vi "DTMF.vi"() -> ()   [LabVIEW 2019]
uses:
  Control 1.ctl
  <vilib>/Waveform/WDTOps.llb/WDT Number of Waveform Samples DBL.vi
  <vilib>/Waveform/WDTOps.llb/WDT Get Waveform Subset DBL.vi
panel:
  out "size(s)":i32
  out "Waveform Chart":dynamicdata(graph)
  in  "stop":bool
  in  "Waveform":waveform(dbl)
  in  "Load File":bool
  out "String":string
  in  "Mode":bool
  out "Collected Signals":dynamicdata(graph)
  out "Signals":dynamicdata(graph)
  in  "stop (F)":bool
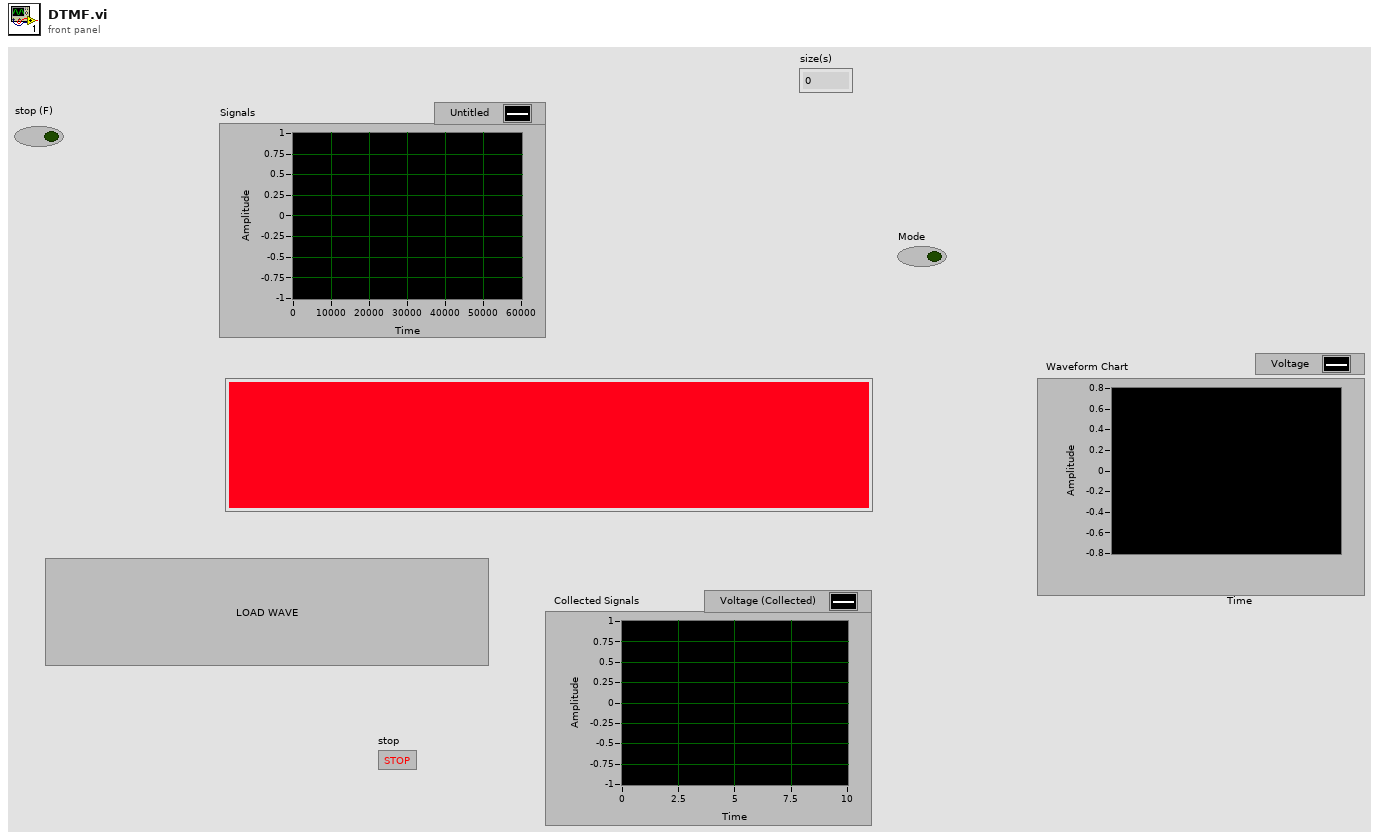
[diagram p1: front panel]
types:
  T1 = typedef "Control 1.ctl" = enum16{"Idle", "Load Image", "Process"}
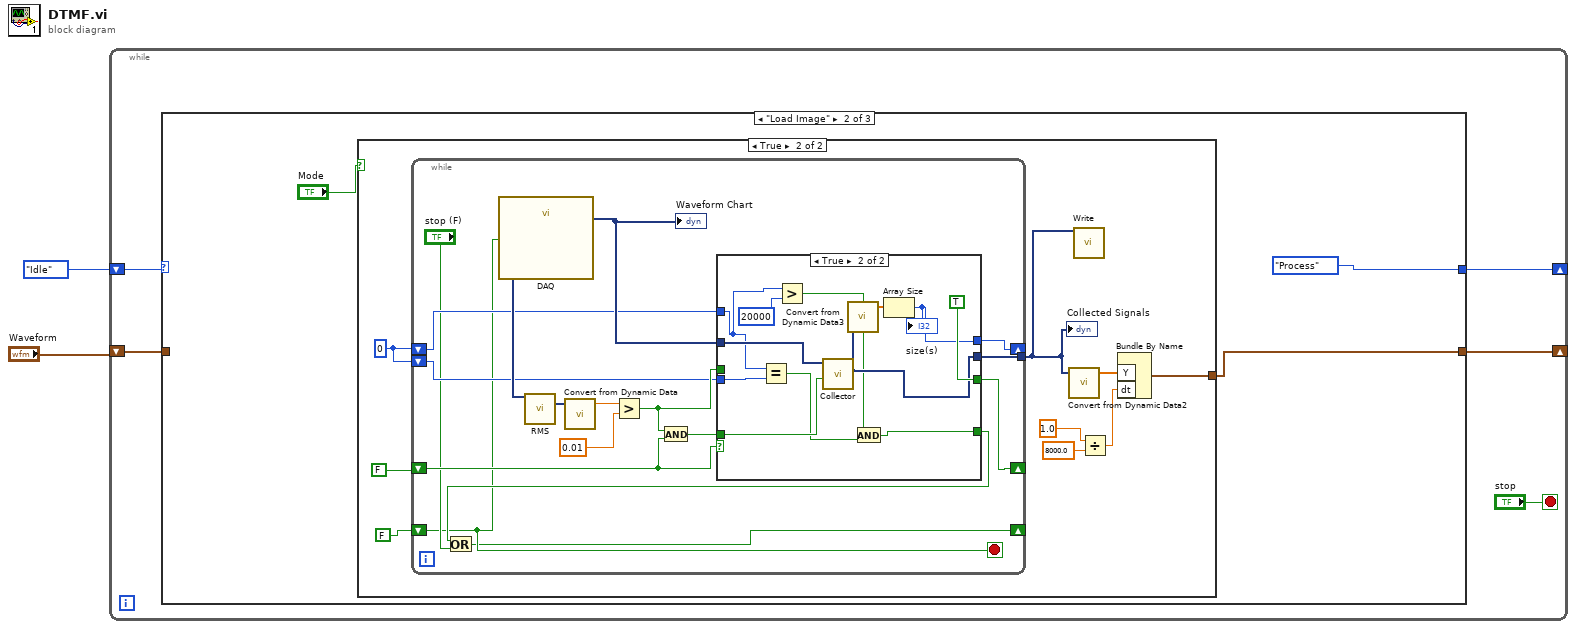
[diagram p0: block diagram]
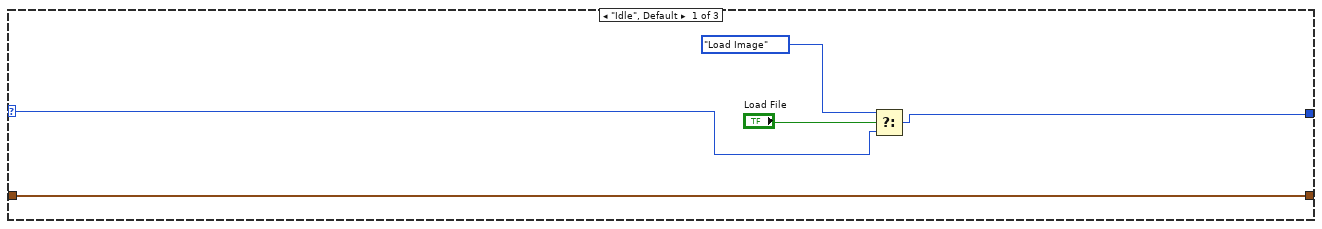
[diagram p2: hidden frame]
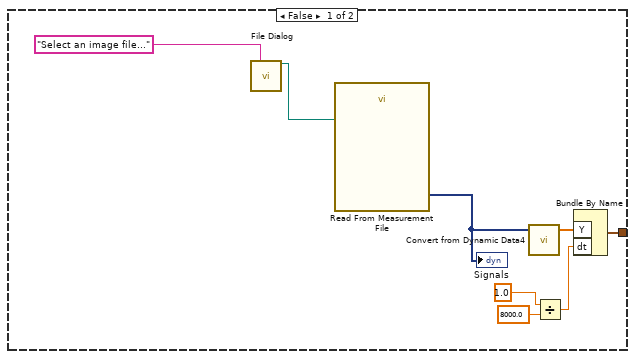
[diagram p3: hidden frame]
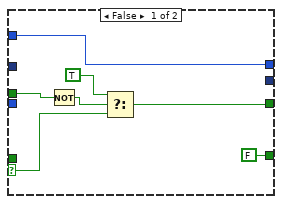
[diagram p4: hidden frame]
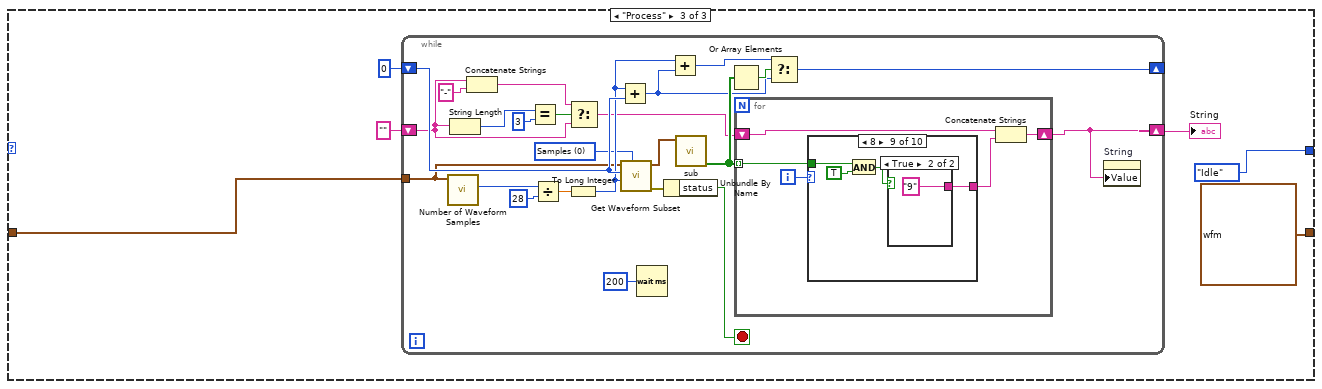
[diagram p5: hidden frame]
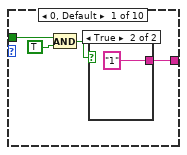
[diagram p6: hidden frame]
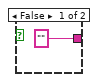
[diagram p7: hidden frame]
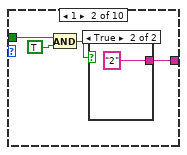
[diagram p8: hidden frame]
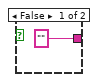
[diagram p9: hidden frame]
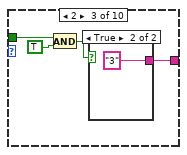
[diagram p10: hidden frame]
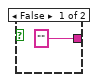
[diagram p11: hidden frame]
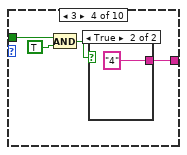
[diagram p12: hidden frame]
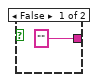
[diagram p13: hidden frame]
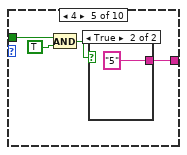
[diagram p14: hidden frame]
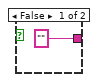
[diagram p15: hidden frame]
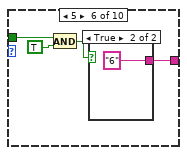
[diagram p16: hidden frame]
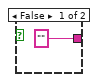
[diagram p17: hidden frame]
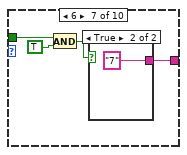
[diagram p18: hidden frame]
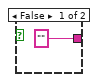
[diagram p19: hidden frame]
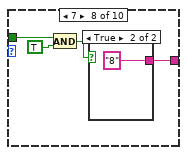
[diagram p20: hidden frame]
diagram:
  n1 = while {
    shift-right: [w6] -> _
    shift-left: Control_1."Idle" -> [w7]
    shift-right: [w4] -> _
    shift-left: "Waveform" -> [w5]
    stop <- "stop" stop-if-true
    n2 = case shown="\"Load Image\"" w7 {
      selector: w7 -> [w11 _ _]
      tunnel: [w9 Control_1."Process" Control_1."Idle"] -> w6
      tunnel: w5 -> [w8 _ w70]
      tunnel: [w8 w14 waveform(dbl) {"t0"=timestamp(0 s since 1904-01-01), "dt"=1.0, "Y"=[]} ("Waveform")] -> w4
      frame "Idle", Default {
        n3 = Select(t=Control_1."Load Image", s="Load File", f=w11) -> (s? t:f=w9:T1)
      }
      frame "Load Image" {
        n4 = case shown="True" "Mode" {
          tunnel: [w18 w28] -> w14
          frame False {
            n5 = call "File Dialog"("prompt"="Select an image file...") -> ("selected path"=w16:path)  [unwired: 6 in, 8 out]
            n6 = call "Read From Measurement File"("Filename"=w16) -> ("Signals"=w23:dynamicdata)  [unwired: 5 in, 5 out]
            "Signals" <- w23
            n7 = call "Convert from Dynamic Data4"("Dynamic Data Type"=w23) -> ("Array"=w22:dbl[])  [unwired: 3 in]
            n8 = Divide(x=1.0, y=8000.0) -> (x/y=w19:dbl)
            n9 = Bundle By Name("Y"=w22, "dt"=w19) -> (w18:waveform(dbl))  [unwired: 1 in]
          }
          frame True {
            w25 = 0
            n10 = while {
              tunnel: [w44] -> w27
              shift-right: [w43] -> _
              shift-left: FALSE -> [w40]
              shift-right: [w36] -> _
              shift-left: w25 -> [w38]
              shift-left: w25 -> [w37]
              shift-right: [w33] -> _
              shift-left: FALSE -> [w34]
              stop <- w34 stop-if-true
              n11 = call "DAQ"("stop (F)"=w34) -> ("data"=w45:dynamicdata)  [unwired: 15 in, 3 out]
              "Waveform Chart" <- w45
              n12 = call "RMS"("Signals"=w45) -> ("RMS"=w48:dynamicdata)  [unwired: 13 in, 1 out]
              n13 = call "Convert from Dynamic Data"("Dynamic Data Type"=w48) -> ("Scalar"=w46:dbl)  [unwired: 3 in]
              n14 = Greater?(x=w46, y=0.01) -> (0:w41:bool)
              n15 = And(x=w41, y=w40) -> (x .and. y?=w39:bool)
              n16 = case shown="True" w40 {
                selector: w40 -> [w55 _]
                tunnel: w41 -> [w51 _]
                tunnel: w45 -> [_ w67]
                tunnel: [_ w64] -> w44
                tunnel: [w53 TRUE ("t")] -> w43
                tunnel: [FALSE w58] -> w42
                tunnel: w39 -> [_ w65]
                tunnel: w38 -> [w49 w57]
                tunnel: w37 -> [_ w60]
                tunnel: [w49 w56] -> w36
                frame False {
                  n17 = Not(x=w51) -> (.not. x?=w50:bool)
                  n18 = Select(t=TRUE, s=w50, f=w55) -> (s? t:f=w53:bool)
                }
                frame True {
                  n19 = Equal?(x=w57, y=w60) -> (x = y?=w59:bool)
                  n20 = Greater?(x=w57, y=20000) -> (0:w61:bool)
                  n21 = call "Collector"("Enable"=w65, "Signals"=w67) -> ("Collected Signals"=w64:dynamicdata)  [unwired: 8 in, 1 out]
                  n22 = call "Convert from Dynamic Data3"("Dynamic Data Type"=w64) -> ("Array"=w63:dbl[])  [unwired: 3 in]
                  n23 = And(x=w61, y=w59) -> (x .and. y?=w58:bool)
                  n24 = Array Size(array=w63) -> (size(s)=w56:i32)
                  "size(s)" <- w56
                }
              }
              n25 = Or(x=w42, y="stop (F)") -> (x .or. y?=w33:bool)
            }
            "Collected Signals" <- w27
            n26 = call "Convert from Dynamic Data2"("Dynamic Data Type"=w27) -> ("Array"=w32:dbl[])  [unwired: 3 in]
            n27 = call "Write"("Signals"=w27) -> ()  [unwired: 16 in, 3 out]
            n28 = Divide(x=1.0, y=8000.0) -> (x/y=w29:dbl)
            n29 = Bundle By Name("Y"=w32, "dt"=w29) -> (w28:waveform(dbl))  [unwired: 1 in]
          }
        }
      }
      frame "Process" {
        n30 = while {
          tunnel: w70 -> [w77]
          shift-right: [w91] -> _
          shift-left: 0 -> [w97]
          shift-right: [w75] -> w73
          shift-left: "" -> [w79]
          stop <- w95 stop-if-true
          w83 = u16 0 items=["Samples", "Relative Time"] ("start/duration format")
          n31 = call-poly <vilib>:"Number of Waveform Samples.vi"("waveform in"=w77) -> ("number of samples"=w76:i32)  [unwired: 8 in, 2 out]
          n32 = String Length(string=w79) -> (length=w85:i32)
          n33 = Concatenate Strings(w79, "-" ("string")) -> (w80:string)
          n34 = Equal?(x=w85, y=3) -> (x = y?=w82:bool)
          n35 = Divide(x=w76, y=28) -> (x/y=w87:dbl)
          n36 = To Long Integer(number=w87) -> (32bit integer=w86:i32)
          n37 = Select(t=w80, s=w82, f=w79) -> (s? t:f=w81:string)
          n38 = Add(x=w86, y=w97) -> (x+y=w90:i32)
          n39 = call-poly <vilib>:"Get Waveform Subset.vi"("start/duration format"=w83, "duration"=w86, "start samples/time"=w97, "waveform in"=w77) -> ("error out"=w96:errorcluster, "waveform out"=w94:waveform(dbl))  [unwired: 2 in, 2 out]
          n40 = Wait (ms)(milliseconds to wait=u32 200) -> ()  [unwired: 1 out]
          n41 = Unbundle By Name(w96) -> ("status"=w95:bool)
          n42 = Add(x=w86, y=w90) -> (x+y=w89:i32)
          n43 = call "sub.vi"("Waveform Graph 8"=w94) -> ("appended array"=w93:bool[])  [unwired: 9 in, 1 out]
          n44 = Or Array Elements(Boolean array=w93) -> (logical OR=w92:bool)
          n45 = for {
            tunnel: w93 -> [w101] mode=indexing
            shift-right: [w98] -> w75
            shift-left: w81 -> [w100]
            i -> [w102]
            n46 = case shown="8" w102 {
              tunnel: w101 -> [w106 w112 w118 w124 w130 w136 w142 w148 w154 w160]
              tunnel: [w103 w109 w115 w121 w127 w133 w139 w145 w151 w157] -> w99
              frame 0, Default {
                n47 = And(x=w106, y=TRUE) -> (x .and. y?=w104:bool)
                n48 = case shown="True" w104 {
                  tunnel: ["" "1"] -> w103
                  frame False {
                  }
                  frame True {
                  }
                }
              }
              frame 1 {
                n49 = And(x=w112, y=TRUE) -> (x .and. y?=w110:bool)
                n50 = case shown="True" w110 {
                  tunnel: ["" "2"] -> w109
                  frame False {
                  }
                  frame True {
                  }
                }
              }
              frame 2 {
                n51 = And(x=w118, y=TRUE) -> (x .and. y?=w116:bool)
                n52 = case shown="True" w116 {
                  tunnel: ["" "3"] -> w115
                  frame False {
                  }
                  frame True {
                  }
                }
              }
              frame 3 {
                n53 = And(x=w124, y=TRUE) -> (x .and. y?=w122:bool)
                n54 = case shown="True" w122 {
                  tunnel: ["" "4"] -> w121
                  frame False {
                  }
                  frame True {
                  }
                }
              }
              frame 4 {
                n55 = And(x=w130, y=TRUE) -> (x .and. y?=w128:bool)
                n56 = case shown="True" w128 {
                  tunnel: ["" "5"] -> w127
                  frame False {
                  }
                  frame True {
                  }
                }
              }
              frame 5 {
                n57 = And(x=w136, y=TRUE) -> (x .and. y?=w134:bool)
                n58 = case shown="True" w134 {
                  tunnel: ["" "6"] -> w133
                  frame False {
                  }
                  frame True {
                  }
                }
              }
              frame 6 {
                n59 = And(x=w142, y=TRUE) -> (x .and. y?=w140:bool)
                n60 = case shown="True" w140 {
                  tunnel: ["" "7"] -> w139
                  frame False {
                  }
                  frame True {
                  }
                }
              }
              frame 7 {
                n61 = And(x=w148, y=TRUE) -> (x .and. y?=w146:bool)
                n62 = case shown="True" w146 {
                  tunnel: ["" "8"] -> w145
                  frame False {
                  }
                  frame True {
                  }
                }
              }
              frame 8 {
                n63 = And(x=w154, y=TRUE) -> (x .and. y?=w152:bool)
                n64 = case shown="True" w152 {
                  tunnel: ["" "9"] -> w151
                  frame False {
                  }
                  frame True {
                  }
                }
              }
              frame 9 {
                n65 = And(x=w160, y=TRUE) -> (x .and. y?=w158:bool)
                n66 = case shown="True" w158 {
                  tunnel: ["" "0"] -> w157
                  frame False {
                  }
                  frame True {
                  }
                }
              }
            }
            n67 = Concatenate Strings(w100, w99) -> (w98:string)
          }
          n68 = Select(t=w89, s=w92, f=w90) -> (s? t:f=w91:i32)
          n69 = property on="String" class="Str"("Value"=w75) -> ()  [unwired: 2 in, 2 out]
        }
        "String" <- w73
      }
    }
  }
